vi "Actor Core.vi"(8 "error in":errorcluster, 11 "Actor_Log in":refnum<class "Actor_Log.lvclass">) -> (0 "error out":errorcluster, 3 "Actor out":refnum<class "Actor.lvclass">)   [LabVIEW 2020, in "Library Core.lvlib" / "Actor_Log.lvlib" / "Actor_Log.lvclass"]
doc: "(<B>Filename</B>: Actor Framework.lvlib:Actor.lvclass:Actor Core.vi)\n\nReceives messages to the actor, reacts to them, and initiates any error handling that may shut the actor down.\n\nDescendant classes may override this VI to append parallel tasks for the actor to complete while it handles messages. Overrides use the Call Parent Method node."
uses:
  Actor_Log.lvclass
  <vilib>/ActorFramework/Actor/Actor.lvclass
  Actor_Log.lvclass/Actor_Log.ctl
  C:/Program Files (x86)/National Instruments/LabVIEW 2020/vi.lib/ActorFramework/Actor/Actor.lvclass
  <vilib>/ActorFramework/Stop Msg/Stop Msg.lvclass
panel:
  out "Logs":string
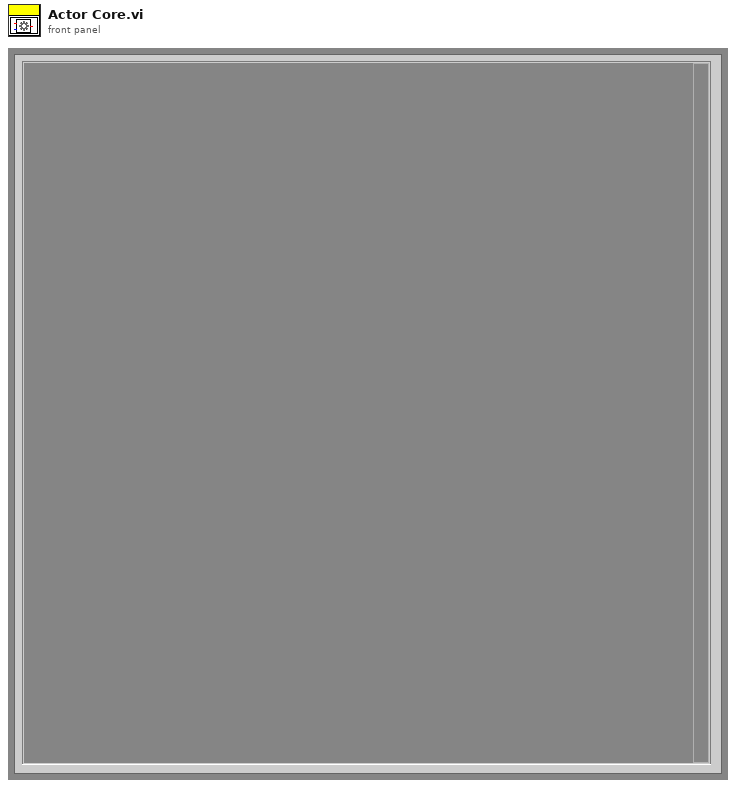
[diagram p1: front panel]
types:
  T1 = enum32{"Invalid", "Standard", "Closed", "Hidden", "Minimized", "Maximized"}
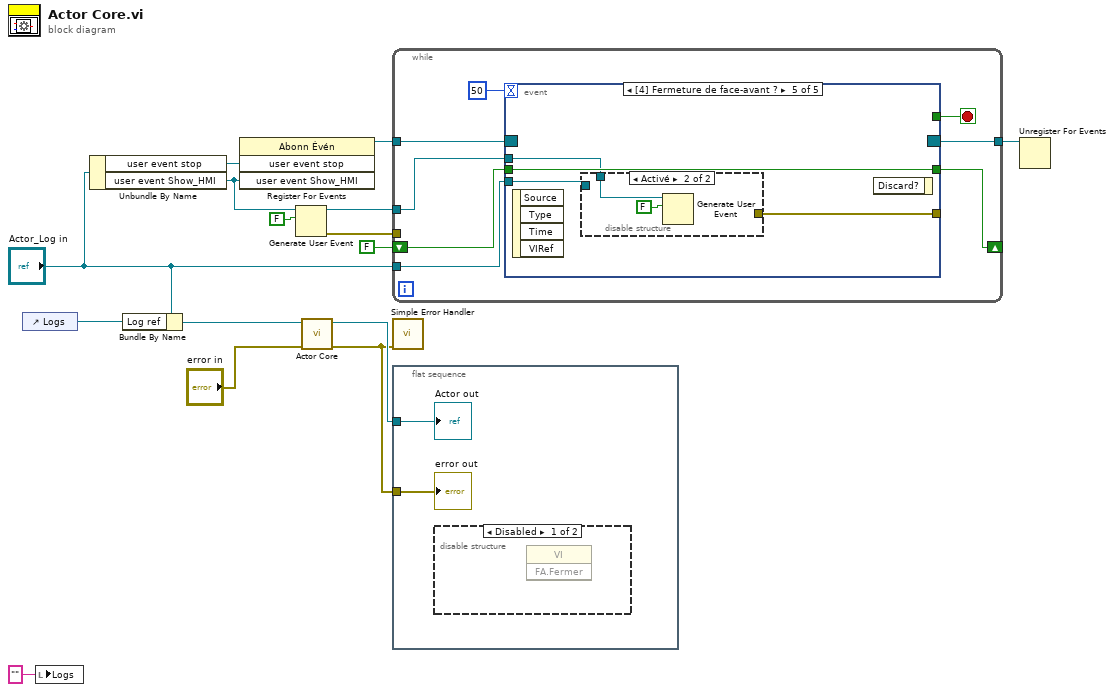
[diagram p0: block diagram]
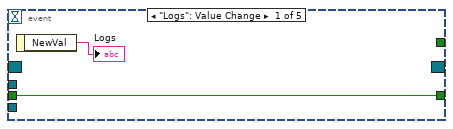
[diagram p3: hidden frame]
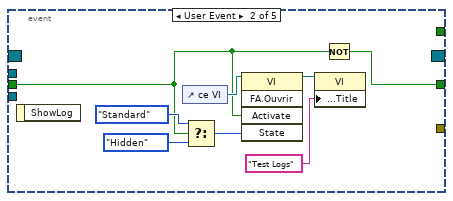
[diagram p4: hidden frame]
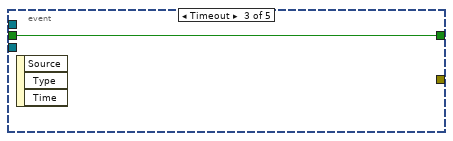
[diagram p5: hidden frame]
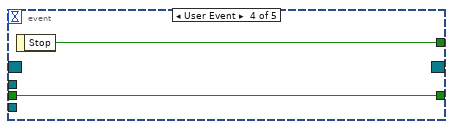
[diagram p6: hidden frame]
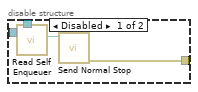
[diagram p7: hidden frame]
diagram:
  n1 = control-ref of="Logs"() -> (w12:refnum<vi>)
  n2 = local write "Logs"("" ("Logs")) -> ()
  n3 = Unbundle By Name("Actor_Log in") -> ("user event stop"=w11:refnum<user-event>, "user event Show_HMI"=w2:refnum<user-event>)
  n4 = Bundle By Name(cluster="Actor_Log in", "Log ref"=w12) -> (w13:refnum<class "Actor_Log.lvclass">)
  n5 = register-events(w11, w2) -> (reference out=w10:refnum<event-registration>)  [unwired: 2 in, 1 out]
  n6 = Generate User Event(user event=w2, event data cluster=FALSE ("données d'événement")) -> (user event out=w1:refnum<user-event>, error out=w3:errorcluster)  [unwired: 2 in]
  n7 = call-parent "Actor Core.vi"("error in"="error in", "Actor in"=w13) -> ("error out"=w7:errorcluster, "Actor out"=w15:refnum<class "Actor.lvclass">)  [unwired: 8 in]
  n8 = while {
    tunnel: w10 -> [w23]
    tunnel: [w22] -> w9
    tunnel: "Actor_Log in" -> [w20]
    shift-right: [w18] -> _
    shift-left: FALSE ("Activer ?") -> [w19]
    tunnel: w3 -> [_]
    tunnel: w1 -> [w16]
    stop <- w21 stop-if-true
    n9 = event shown="[4] Fermeture de face-avant ?" {
      selector: w23 -> [_ _ _ _ _]
      dyn-events: [_ _ _ _ _] -> w22
      timeout: 50 -> [_ _ _ _ _]
      tunnel: [_ _ _ w36 _] -> w21
      tunnel: w20 -> [_ _ _ _ w40]
      tunnel: w19 -> [w24 w29 w34 w35 w39]
      tunnel: [w24 w28 w34 w35 w39] -> w18
      tunnel: [_ _ _ _ w38] -> _
      tunnel: w16 -> [_ _ _ _ w37]
      event "Logs": Value Change {
        n10 = event-data() -> ("NewVal"=→"Logs":string)  [unwired: 1 in]
      }
      event User Event {
        n11 = event-data() -> ()  [unwired: 1 in, 1 out]
        n12 = control-ref of="ce VI"() -> (w33:refnum<vi>)
        n13 = Select(t=T1."Standard" ("État"), s=w29, f=T1."Hidden" ("État")) -> (s? t:f=w30:T1)
        n14 = invoke class="VI" method="FA.Ouvrir"(reference=w33, "Activate"=w29, "State"=w30) -> (reference out=w27:refnum<vi>)  [unwired: 2 in, 4 out]
        n15 = property class="VI"(reference=w27, "Front Panel.Title"="Test Logs" ("Fenêtre face-avant:Titre")) -> ()  [unwired: 1 in, 2 out]
        n16 = Not(x=w29) -> (.not. x?=w28:bool)
      }
      event Timeout {
        n17 = event-data() -> ()  [unwired: 1 in, 3 out]
      }
      event User Event {
        n18 = event-data() -> ("Stop"=w36:bool)  [unwired: 1 in]
      }
      event Panel Close? {
        n19 = event-data() -> ()  [unwired: 1 in, 4 out]
        n20 = disable-structure shown="Activé" {
          disable-tunnel: w40 -> [w42 _]
          disable-tunnel: [w41 _] -> w38
          disable-tunnel: w37 -> [_ w44]
          frame Disabled {
            n21 = call <vilib>:"Read Self Enqueuer.vi"("Actor"=w42) -> ("Self Enqueuer"=w43:refnum<class "Message Enqueuer.lvclass">)  [unwired: 10 in]
            n22 = call <vilib>:"Send Normal Stop.vi"("Message Enqueuer"=w43) -> ("error out"=w41:errorcluster)  [unwired: 10 in]
          }
          frame Enabled {
            n23 = Generate User Event(user event=w44, event data cluster=FALSE ("données d'événement")) -> ()  [unwired: 2 in, 2 out]
          }
        }
        n24 = event-data() -> ()  [unwired: 2 in, 1 out]
      }
    }
  }
  n25 = call <vilib>:"Simple Error Handler.vi"("error in (no error)"=w7) -> ()  [unwired: 4 in, 5 out]
  n26 = flat-sequence {
    tunnel: w7 -> [w47]
    tunnel: w15 -> [w46]
    frame #0 {
      n27 = disable-structure shown="Activé" {
        frame Disabled {
          n28 = invoke class="VI" method="FA.Fermer"() -> ()  [unwired: 3 in, 3 out]
        }
        frame Enabled {
        }
      }
      "error out" <- w47
      "Actor out" <- w46
    }
  }
  n29 = Unregister For Events(event registration refnum=w9) -> ()  [unwired: 1 in, 1 out]
